vi "UR Server 2.vi"() -> ()   [LabVIEW 2019]
panel:
  in  "stop":bool
  out "size(s)":i32
  out "data":string
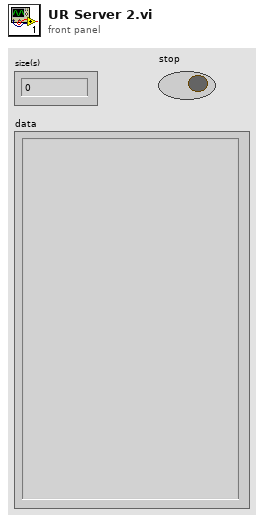
[diagram p1: front panel]
types:
  T1 = enum16{"Standard", "Buffered", "CRLF", "Immediate"}
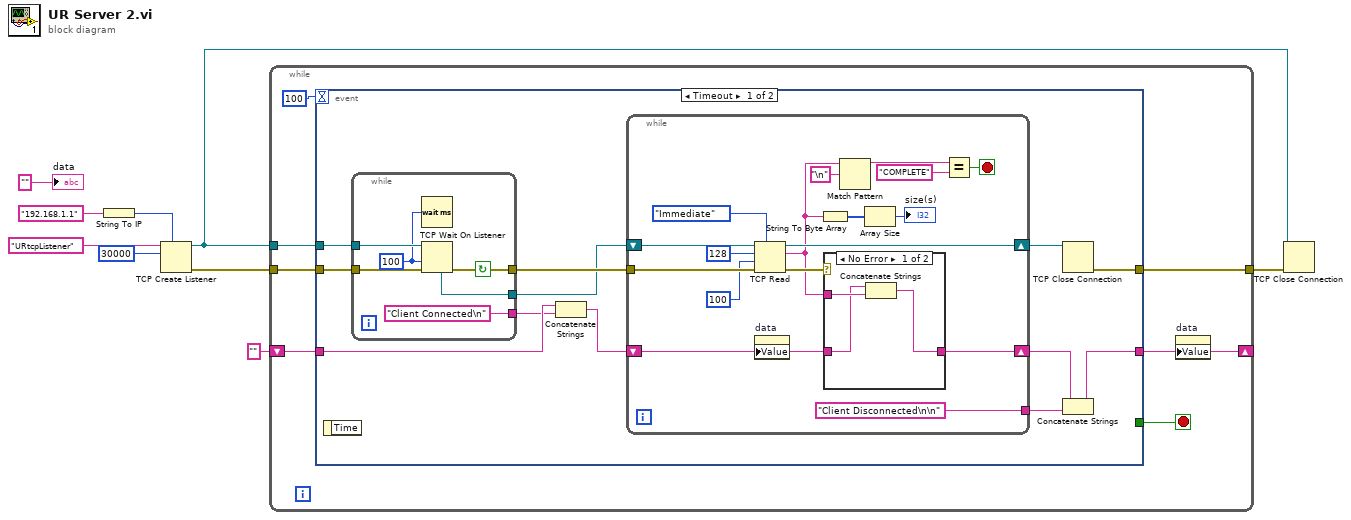
[diagram p0: block diagram]
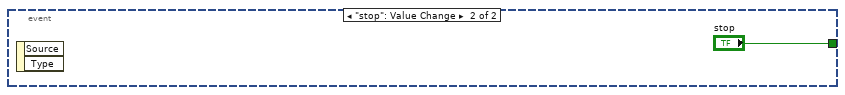
[diagram p3: hidden frame]
diagram:
  n1 = String To IP(1:"192.168.1.1" ("name")) -> (0:w7:u32)
  n2 = TCP Create Listener(7:w7, 10:u16 30000 ("remote port or service name"), 11:"URtcpListener" ("service name")) -> (0:w5:errorcluster, 3:w4:refnum<k5>)  [unwired: 2 in, 1 out]
  n3 = while {
    tunnel: w5 -> [w16]
    tunnel: w4 -> [w15]
    tunnel: [w14] -> w2
    shift-right: [w10] -> _
    shift-left: "" -> [w11]
    stop <- w12 stop-if-true
    n4 = event shown="[0] Timeout" {
      selector: _ -> [_ _]
      dyn-events: _ -> [_ _]
      timeout: 100 -> [_ _]
      tunnel: w16 -> [w28 _]
      tunnel: w15 -> [w27 _]
      tunnel: [w23 _] -> w14
      tunnel: [_ "stop"] -> w12
      tunnel: [w18 _] -> w10
      tunnel: w11 -> [w22 _]
      event Timeout {
        n5 = event-data() -> ()  [unwired: 1 in, 1 out]
        n6 = while {
          tunnel: w28 -> [w54]
          tunnel: [w52] -> w26
          tunnel: [w51] -> w25
          tunnel: w27 -> [w55]
          tunnel: ["Client Connected\n"] -> w20
          stop <- w52 continue-if-true
          w53 = 100 ("timeout ms (wait forever: -1)")
          n7 = Wait (ms)(milliseconds to wait=w53) -> ()  [unwired: 1 out]
          n8 = TCP Wait On Listener(8:w54, 9:w53, 11:w55) -> (0:w52:errorcluster, 4:w51:refnum<k5>)  [unwired: 1 in, 3 out]
        }
        n9 = Concatenate Strings(w22, w20) -> (w21:string)
        n10 = while {
          shift-right: [w45] -> w24
          shift-left: w25 -> [w43]
          tunnel: w26 -> [w44]
          shift-right: [w30] -> w19
          shift-left: w21 -> [w31]
          tunnel: ["Client Disconnected\n\n"] -> w17
          stop <- w33 stop-if-true
          n11 = TCP Read(connection ID=w43, bytes to read=128, error in (no error)=w44, 7:T1."Immediate" ("mode (standard)"), 9:100 ("timeout ms (25000)")) -> (connection ID out=w45:refnum<k5>, data out=w36:string, error out=w42:errorcluster)
          n12 = property on="data" class="Str"("Value"=w31) -> ()  [unwired: 2 in, 2 out]
          n13 = String To Byte Array(string=w36) -> (unsigned byte array=w38:u8[])
          n14 = case shown="No Error" w42 {
            tunnel: w36 -> [w48 _]
            tunnel: [w47 w49] -> w30
            tunnel: w31 -> [w46 w49]
            frame No Error {
              n15 = Concatenate Strings(w46, w48) -> (w47:string)
            }
            frame Error {
            }
          }
          n16 = Match Pattern(string=w36, regular expression="\n") -> (before substring=w34:string)  [unwired: 1 in, 3 out]
          n17 = Array Size(array=w38) -> (size(s)=→"size(s)":i32)
          n18 = Equal?(x=w34, y="COMPLETE") -> (x = y?=w33:bool)
        }
        n19 = TCP Close Connection(connection ID=w24) -> (error out=w23:errorcluster)  [unwired: 2 in, 1 out]
        n20 = Concatenate Strings(w19, w17) -> (w18:string)
      }
      event "stop": Value Change {
        n21 = event-data() -> ()  [unwired: 1 in, 2 out]
      }
    }
    n22 = property on="data" class="Str"("Value"=w10) -> ()  [unwired: 2 in, 2 out]
  }
  n23 = TCP Close Connection(connection ID=w4, error in (no error)=w2) -> ()  [unwired: 1 in, 2 out]
  "data" <- "" ("data out")
